vi "Labview_USB_I2C_AM2321B.vi"() -> ()   [LabVIEW 2010]
uses:
  Labview_USB_I2C_AM2321B/lib/labview_32bit/ControlI2C/Ginkgo_Driver.dll
panel:
  out "error out":errorcluster
  in  "stop":bool
  in  "OK":bool
  out "Oscillogram":dbl[][](graph)
  in  "Channel Index":u16(ring) items=["0", "1"]
  in  "Speed":u32(ring)=800000 items=["800Kbps"=800000, "400Kbps"=400000, "200Kbps"=200000, "100Kbps"=100000, "50Kbps"=50000]
  in  "Device Index":i32(ring) items=["0", "1", "2", "3", "4", "5", "6", "7", "8", "9"]
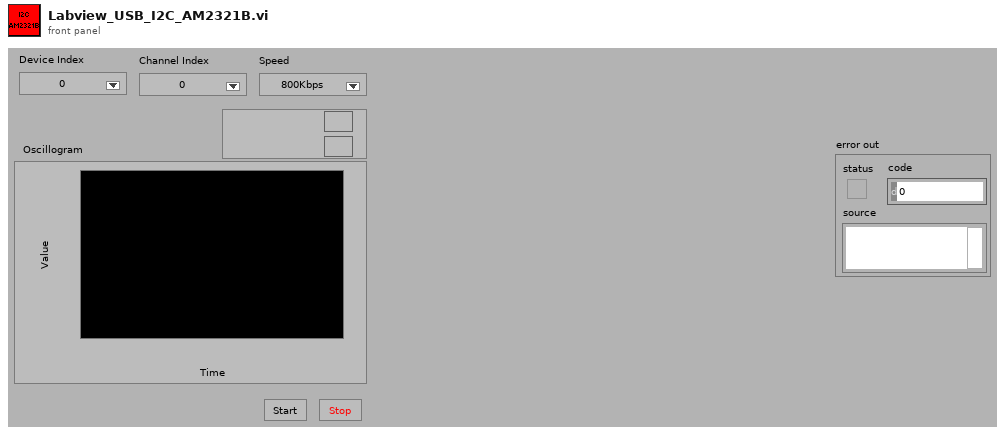
[diagram p1: front panel]
types:
  T1 = enum16{"Init", "ScanDevice", "OpenDevice", "InitDevice", "Read data", "Idel", "Close", "Error"}
  T2 = cluster{"MasterMode":u8, "ControlMode":u8, "AddrType":u8, "SubAddrWidth":u8, "Addr":u16, "@dummy control@":i8, "@dummy control@":i8, "ClockSpeed":u32}
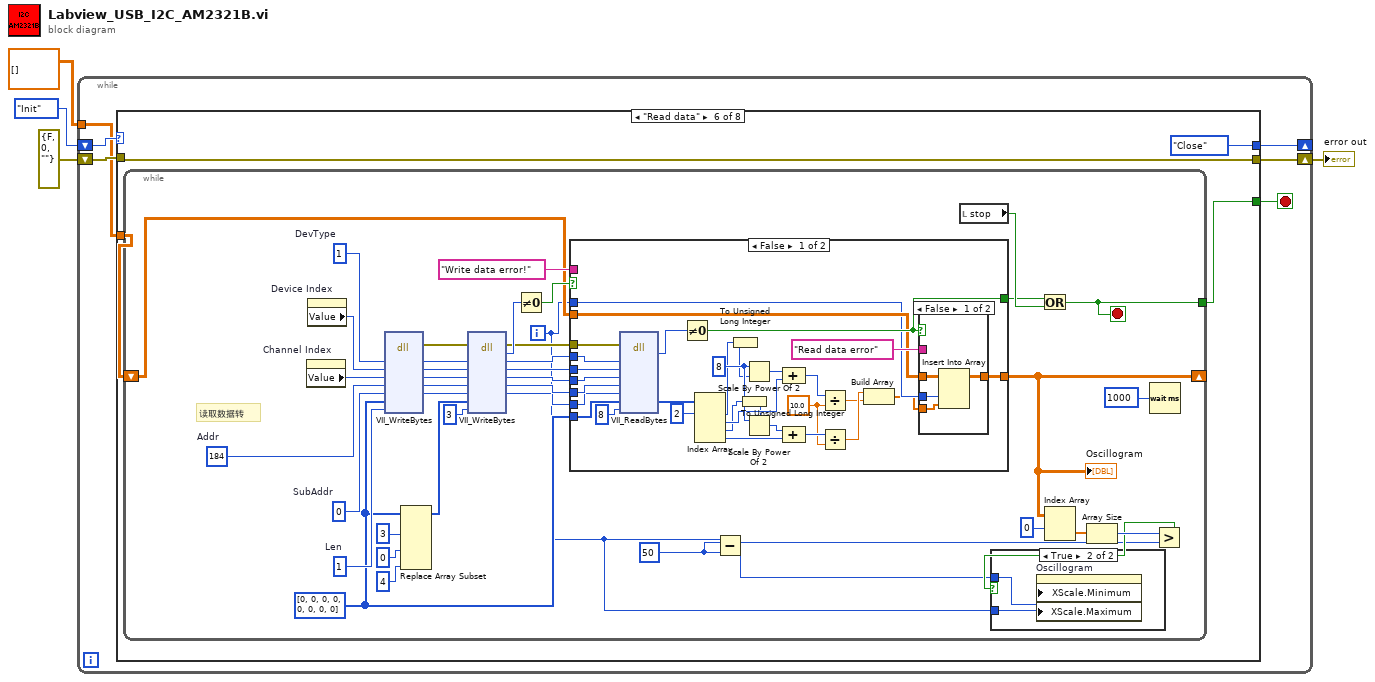
[diagram p0: block diagram]
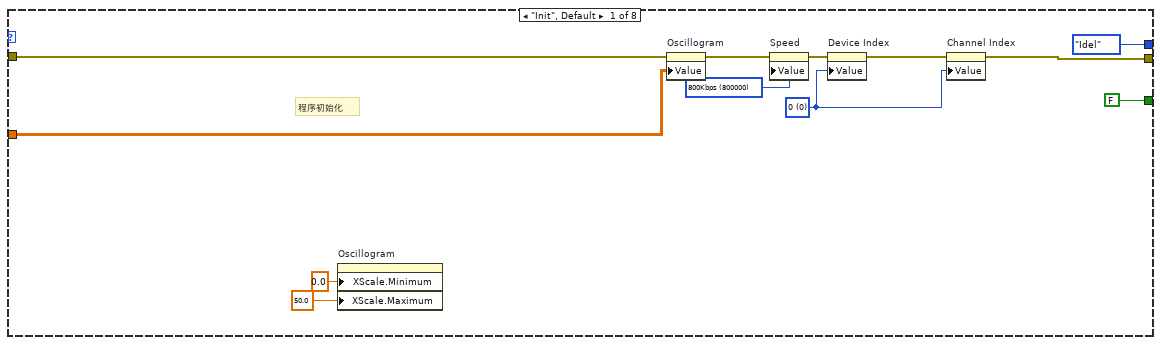
[diagram p2: hidden frame]
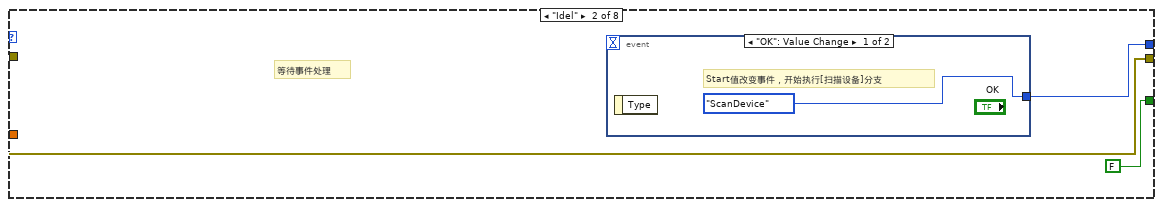
[diagram p3: hidden frame]
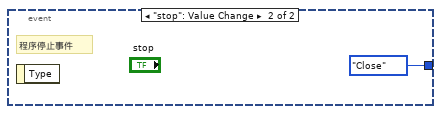
[diagram p4: hidden frame]
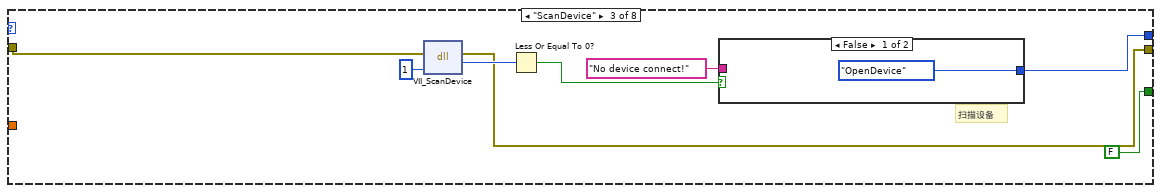
[diagram p5: hidden frame]
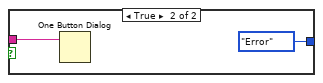
[diagram p6: hidden frame]
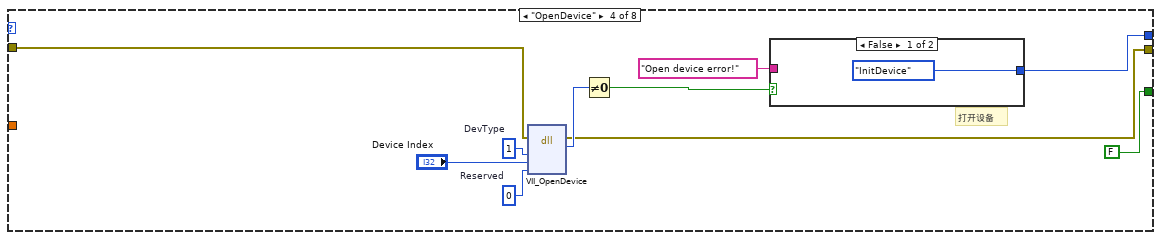
[diagram p7: hidden frame]
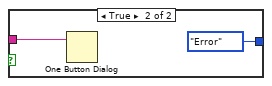
[diagram p8: hidden frame]
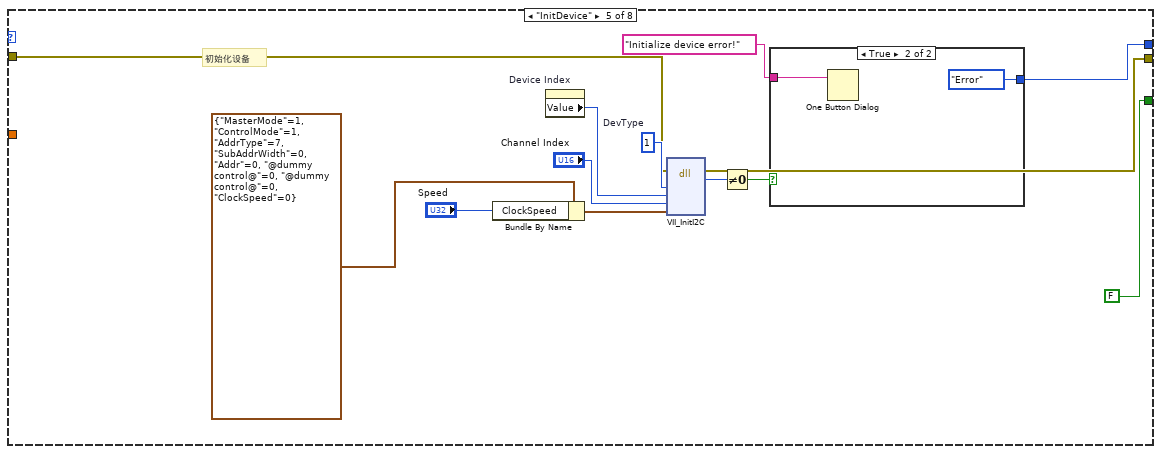
[diagram p9: hidden frame]
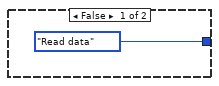
[diagram p10: hidden frame]
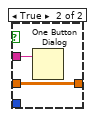
[diagram p12: hidden frame]
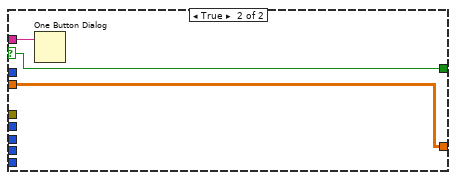
[diagram p13: hidden frame]
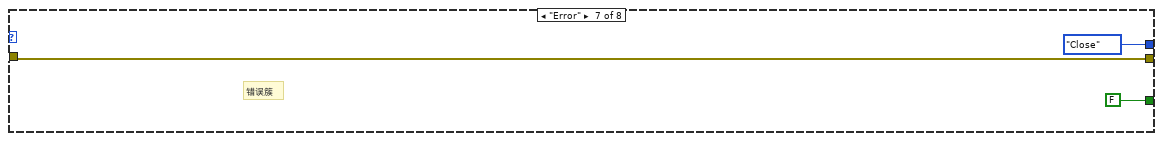
[diagram p14: hidden frame]
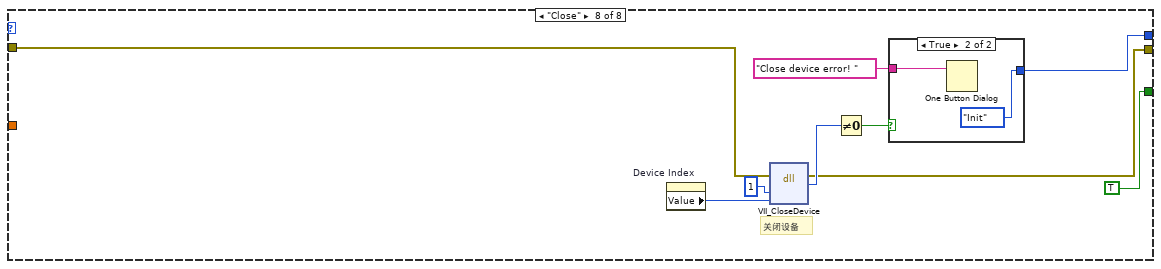
[diagram p15: hidden frame]
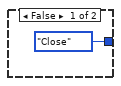
[diagram p16: hidden frame]
diagram:
  n1 = while {
    shift-right: [w10] -> _
    shift-left: T1."Init" ("Enum") -> [w9]
    shift-right: [w7] -> w2
    shift-left: errorcluster {"status"=FALSE, "code"=0, "source"=""} ("error out") -> [w6]
    tunnel: dbl[][] [] -> [w5]
    stop <- w8 stop-if-true
    n2 = case shown="\"Read data\"" w9 {
      tunnel: [T1."Idel" ("Enum") w25 w31 w43 w59 T1."Close" ("Enum") T1."Close" ("Enum") w160] -> w10
      tunnel: [FALSE ("stop") FALSE ("stop") FALSE ("stop") FALSE ("stop") FALSE ("stop") w69 FALSE ("stop") TRUE ("stop")] -> w8
      tunnel: [w19 w24 w29 w40 w53 w71 w155 w157] -> w7
      tunnel: w6 -> [w16 w24 w28 w41 w54 w71 w155 w158]
      tunnel: w5 -> [w17 _ _ _ _ w70 _ _]
      frame "Init", Default {
        w13 = u32 800000 items=["800Kbps"=800000, "400Kbps"=400000, "200Kbps"=200000, "100Kbps"=100000, "50Kbps"=50000] ("Speed")
        w21 = u16 0 items=["0", "1", "2", "3", "4", "5", "6", "7", "8", "9"] ("Device Index")
        # "程序初始化"
        n3 = property on="Oscillogram" class="WFGraph (strict)"("XScale.Minimum"=0.0 ("X Scale.Range:Minimum"), "XScale.Maximum"=50.0 ("X Scale.Range:Maximum")) -> ()  [unwired: 2 in, 2 out]
        n4 = property on="Oscillogram" class="WFGraph (strict)"(error in=w16, "Value"=w17) -> (error out=w15:errorcluster)  [unwired: 1 in, 1 out]
        n5 = property on="Speed" class="Ring (strict)"(error in=w15, "Value"=w13) -> (error out=w18:errorcluster)  [unwired: 1 in, 1 out]
        n6 = property on="Device Index" class="Ring (strict)"(error in=w18, "Value"=w21) -> (error out=w20:errorcluster)  [unwired: 1 in, 1 out]
        n7 = property on="Channel Index" class="Ring (strict)"(error in=w20, "Value"=w21) -> (error out=w19:errorcluster)  [unwired: 1 in, 1 out]
      }
      frame "Idel" {
        # "等待事件处理"
        n8 = event shown="[0] \"OK\": Value Change" {
          selector: _ -> [_ _]
          dyn-events: _ -> [_ _]
          timeout: _ -> [_ _]
          tunnel: [T1."ScanDevice" ("Enum") T1."Close" ("Enum")] -> w25
          event "OK": Value Change {
            # "Start值改变事件，开始执行[扫描设备]分支"
            n9 = event-data() -> ()  [unwired: 1 in, 1 out]
          }
          event "stop": Value Change {
            # "程序停止事件"
            n10 = event-data() -> ()  [unwired: 1 in, 1 out]
          }
        }
      }
      frame "ScanDevice" {
        # "扫描设备"
        n11 = dll-call lib="E:/Project/vt_ginkgo_examples/trunk/Labview/Ginkgo I2C/Labview_USB_I2C_AM2321B/lib/labview_32bit/ControlI2C/Ginkgo_Driver.dll" fn="VII_ScanDevice"(error in=w28, "NeedInit"=u8 1) -> (error out=w29:errorcluster, "return type"=w34:i32)  [unwired: 3 in, 1 out]
        n12 = Less Or Equal To 0?(x=w34) -> (x <= 0?=w33:bool)
        n13 = case shown="False" w33 {
          tunnel: "No device connect!" ("message") -> [_ w38]
          tunnel: [T1."OpenDevice" ("Enum") T1."Error" ("Enum")] -> w31
          frame False {
          }
          frame True {
            n14 = One Button Dialog(message=w38) -> ()  [unwired: 1 in, 1 out]
          }
        }
      }
      frame "OpenDevice" {
        w47 = 0  # Reserved
        w48 = 1  # DevType
        # "打开设备"
        n15 = dll-call lib="E:/Project/vt_ginkgo_examples/trunk/Labview/Ginkgo I2C/Labview_USB_I2C_AM2321B/lib/labview_32bit/ControlI2C/Ginkgo_Driver.*" fn="VII_OpenDevice"(error in=w41, "DevType"=w48, "DevIndex"="Device Index", "Reserved"=w47) -> (error out=w40:errorcluster, "return type"=w45:i32)  [unwired: 5 in, 1 out]
        n16 = Not Equal To 0?(x=w45) -> (x != 0?=w44:bool)
        n17 = case shown="False" w44 {
          tunnel: "Open device error!" ("message") -> [_ w51]
          tunnel: [T1."InitDevice" ("Enum") T1."Error" ("Enum")] -> w43
          frame False {
          }
          frame True {
            n18 = One Button Dialog(message=w51) -> ()  [unwired: 1 in, 1 out]
          }
        }
      }
      frame "InitDevice" {
        w64 = 1  # DevType
        # "初始化设备"
        n19 = Bundle By Name(cluster=T2 {"MasterMode"=1, "ControlMode"=1, "AddrType"=7, "SubAddrWidth"=0, "Addr"=0, "@dummy control@"=0, "@dummy control@"=0, "ClockSpeed"=0} ("pInitConfig"), "ClockSpeed"="Speed") -> (w55:T2)
        n20 = property on="Device Index" class="Ring (strict)"() -> ("Value"=w63:i32)  [unwired: 2 in, 2 out]
        n21 = dll-call lib="E:/Project/vt_ginkgo_examples/trunk/Labview/Ginkgo I2C/Labview_USB_I2C_AM2321B/lib/labview_32bit/ControlI2C/Ginkgo_Driver.dll" fn="VII_InitI2C"(error in=w54, "DevType"=w64, "DevIndex"=w63, "I2CIndex"="Channel Index", "pInitConfig"=w55) -> (error out=w53:errorcluster, "return type"=w61:i32)  [unwired: 6 in, 1 out]
        n22 = Not Equal To 0?(x=w61) -> (x != 0?=w60:bool)
        n23 = case shown="True" w60 {
          tunnel: "Initialize device error!" ("message") -> [_ w67]
          tunnel: [T1."Read data" ("Enum") T1."Error" ("Enum")] -> w59
          frame False {
          }
          frame True {
            n24 = One Button Dialog(message=w67) -> ()  [unwired: 1 in, 1 out]
          }
        }
      }
      frame "Read data" {
        n25 = while {
          shift-right: [w73] -> _
          shift-left: w70 -> [w84]
          tunnel: [w81] -> w69
          i -> [w72]
          stop <- w81 stop-if-true
          w75 = 50 ("y")
          w85 = u8[] [0, 0, 0, 0, 0, 0, 0, 0] ("pWriteData")
          w106 = u16 1  # Len
          w107 = u32 0  # SubAddr
          w108 = u16 184  # Addr
          w110 = 1  # DevType
          # "读取数据转"
          n26 = property on="Channel Index" class="Ring (strict)"() -> ("Value"=w80:u16)  [unwired: 2 in, 2 out]
          n27 = property on="Device Index" class="Ring (strict)"() -> ("Value"=w109:i32)  [unwired: 2 in, 2 out]
          n28 = dll-call lib="E:/Project/vt_ginkgo_examples/trunk/Labview/Ginkgo I2C/Labview_USB_I2C_AM2321B/lib/labview_32bit/ControlI2C/Ginkgo_Driver.dll" fn="VII_WriteBytes"("DevType"=w110, "DevIndex"=w109, "I2CIndex"=w80, "Addr"=w108, "SubAddr"=w107, "pWriteData"=w85, "Len"=w106) -> (error out=w102:errorcluster, "DevType"=w99:i32, "DevIndex"=w98:i32, "I2CIndex"=w97:i32, "Addr"=w96:u16, "SubAddr"=w95:u32)  [unwired: 6 in, 1 out]
          n29 = Replace Array Subset(array=w85, new element #1=u8 3 ("new element/subarray"), new element #2=u8 0 ("new element/subarray"), new element #3=u8 4 ("new element/subarray")) -> (w101:u8[])  [unwired: 3 in]
          n30 = dll-call lib="E:/Project/vt_ginkgo_examples/trunk/Labview/Ginkgo I2C/Labview_USB_I2C_AM2321B/lib/labview_32bit/ControlI2C/Ginkgo_Driver.dll" fn="VII_WriteBytes"(error in=w102, "DevType"=w99, "DevIndex"=w98, "I2CIndex"=w97, "Addr"=w96, "SubAddr"=w95, "pWriteData"=w101, "Len"=u16 3) -> (error out=w91:errorcluster, "return type"=w94:i32, "DevType"=w90:i32, "DevIndex"=w89:i32, "I2CIndex"=w88:i32, "Addr"=w87:u16, "SubAddr"=w86:u32)  [unwired: 4 in, 1 out]
          n31 = Not Equal To 0?(x=w94) -> (x != 0?=w93:bool)
          n32 = case shown="False" w93 {
            selector: w93 -> [_ w152]
            tunnel: "Write data error!" ("message") -> [_ w153]
            tunnel: w91 -> [w144 _]
            tunnel: w90 -> [w143 _]
            tunnel: w89 -> [w142 _]
            tunnel: w88 -> [w141 _]
            tunnel: w87 -> [w140 _]
            tunnel: w86 -> [w139 _]
            tunnel: w85 -> [w137 _]
            tunnel: [w134 w152] -> w82
            tunnel: w72 -> [w122 _]
            tunnel: w84 -> [w123 w151]
            tunnel: [w120 w151] -> w73
            frame False {
              w124 = 10.0 ("y")
              w129 = 8 ("n")
              n33 = dll-call lib="E:/Project/vt_ginkgo_examples/trunk/Labview/Ginkgo I2C/Labview_USB_I2C_AM2321B/lib/labview_32bit/ControlI2C/Ginkgo_Driver.dll" fn="VII_ReadBytes"(error in=w144, "DevType"=w143, "DevIndex"=w142, "I2CIndex"=w141, "Addr"=w140, "SubAddr"=w139, "pReadData"=w137, "Len"=u16 8) -> ("return type"=w135:i32, "pReadData"=w133:u8[])  [unwired: 8 in, 2 out]
              n34 = Not Equal To 0?(x=w135) -> (x != 0?=w134:bool)
              n35 = Index Array(array=w133, index #1=2 ("index")) -> (element #1=w117:u8, element #2=w127:u8, element #3=w115:u8, element #4=w131:u8)  [unwired: 3 in]
              n36 = To Unsigned Long Integer(number=w117) -> (unsigned 32bit integer=w116:u32)
              n37 = To Unsigned Long Integer(number=w115) -> (unsigned 32bit integer=w114:u32)
              n38 = Scale By Power Of 2(n=w129, x=w116) -> (x*2^n=w128:u32)
              n39 = Scale By Power Of 2(n=w129, x=w114) -> (x*2^n=w132:u32)
              n40 = Compound Arithmetic op=ADD(w128, w127) -> (w126:u32)
              n41 = Compound Arithmetic op=ADD(w132, w131) -> (w130:u32)
              n42 = Divide(x=w126, y=w124) -> (x/y=w119:dbl)
              n43 = Divide(x=w130, y=w124) -> (x/y=w125:dbl)
              n44 = Build Array(w125, w119) -> (w121:dbl[])
              n45 = case shown="False" w134 {
                tunnel: "Read data error" ("message") -> [_ w150]
                tunnel: w123 -> [w148 w149]
                tunnel: w122 -> [w147 _]
                tunnel: w121 -> [w146 _]
                tunnel: [w145 w149] -> w120
                frame False {
                  n46 = Insert Into Array(array=w148, index (col)=w147, new element=w146) -> (w145:dbl[][])  [unwired: 1 in]
                }
                frame True {
                  n47 = One Button Dialog(message=w150) -> ()  [unwired: 1 in, 1 out]
                }
              }
            }
            frame True {
              n48 = One Button Dialog(message=w153) -> ()  [unwired: 1 in, 1 out]
            }
          }
          "Oscillogram" <- w73
          n49 = Subtract(x=w72, y=w75) -> (x-y=w74:i32)
          n50 = local read "stop"() -> (w83:bool)
          n51 = Or(x=w82, y=w83) -> (x .or. y?=w81:bool)
          n52 = Index Array(array=w73, index (row)=0) -> (element=w78:dbl[])  [unwired: 1 in]
          n53 = Array Size(array=w78) -> (size(s)=w77:i32)
          n54 = Wait (ms)(milliseconds to wait=u32 1000) -> ()  [unwired: 1 out]
          n55 = Greater?(x=w77, y=w75) -> (0:w76:bool)
          n56 = case shown="True" w76 {
            tunnel: w74 -> [_ w113]
            tunnel: w72 -> [_ w112]
            frame False {
            }
            frame True {
              n57 = property on="Oscillogram" class="WFGraph (strict)"("XScale.Minimum"=w113, "XScale.Maximum"=w112) -> ()  [unwired: 2 in, 2 out]
            }
          }
        }
      }
      frame "Error" {
        # "错误簇"
      }
      frame "Close" {
        # "关闭设备"
        n58 = property on="Device Index" class="Ring (strict)"() -> ("Value"=w165:i32)  [unwired: 2 in, 2 out]
        n59 = dll-call lib="E:/Project/vt_ginkgo_examples/trunk/Labview/Ginkgo I2C/Labview_USB_I2C_AM2321B/lib/labview_32bit/ControlI2C/Ginkgo_Driver.dll" fn="VII_CloseDevice"(error in=w158, "DevType"=1, "DevIndex"=w165) -> (error out=w157:errorcluster, "return type"=w162:i32)  [unwired: 4 in, 1 out]
        n60 = Not Equal To 0?(x=w162) -> (x != 0?=w161:bool)
        n61 = case shown="True" w161 {
          tunnel: "Close device error! " ("message") -> [_ w168]
          tunnel: [T1."Close" ("Enum") T1."Init" ("Enum")] -> w160
          frame False {
          }
          frame True {
            n62 = One Button Dialog(message=w168) -> ()  [unwired: 1 in, 1 out]
          }
        }
      }
    }
  }
  "error out" <- w2
